vi "Close.vi"(8 "error in (no error)":errorcluster, 11 "KNF Settings":T1={"VISA resource name"="", "Simulated?"=TRUE}) -> (0 "error out":errorcluster, 1 "Connection Error":bool, 3 "KNF Settings":T1={"VISA resource name"="", "Simulated?"=TRUE})   [LabVIEW 2018, in "KNF SIMDOS.lvlib"]
uses:
  KNF SIMDOS.lvlib
  Settings Cluster plus SIMDOS.ctl
  <vilib>/KNF LAB/Driver S/Lvlib/SIMLAB_driver_lvclass/SIMLAB_driver.lvclass
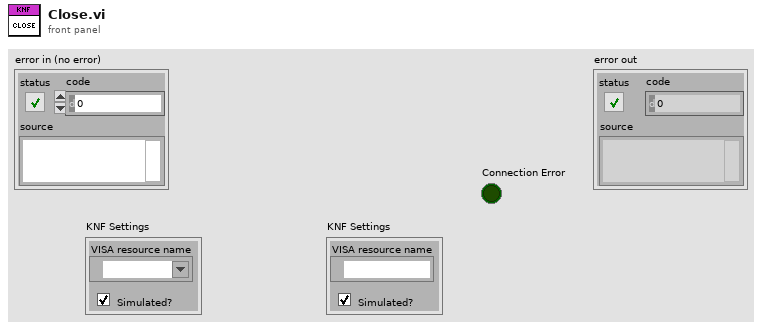
[diagram p1: front panel]
types:
  T1 = typedef "KNF SIMDOS.lvlib/Settings Cluster plus SIMDOS.ctl" = cluster{"VISA resource name":refnum<visa-resource-name>, "Simulated?":bool}
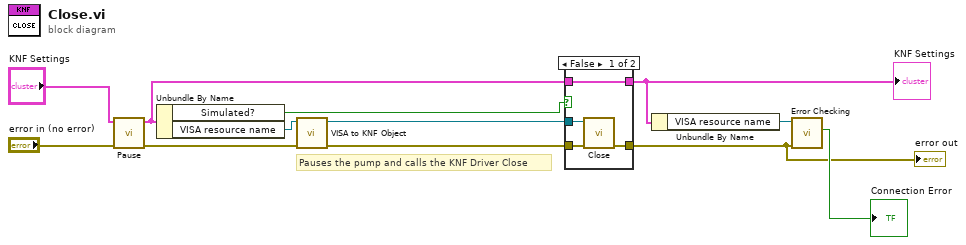
[diagram p0: block diagram]
diagram:
  # "Pauses the pump and calls the KNF Driver Close"
  n1 = call "Pause.vi"("error in (no error)"="error in (no error)", "KNF Settings"="KNF Settings") -> ("error out"=w7:errorcluster, "KNF Settings"=w5:T1)  [unwired: 7 in, 1 out]
  n2 = Unbundle By Name(w5) -> ("Simulated?"=w12:bool, "VISA resource name"=w11:refnum<visa-resource-name>)
  n3 = call "VISA to KNF Object.vi"("error in (no error)"=w7, "VISA resource name"=w11) -> ("error out"=w9:errorcluster, "SIMDOS out"=w10:refnum<class "SIMLAB_driver.lvclass">)  [unwired: 8 in]
  n4 = case shown="False" w12 {
    tunnel: [w15 w18] -> w2
    tunnel: w5 -> [w15 w18]
    tunnel: [w14 w17] -> w3
    tunnel: w9 -> [w13 w17]
    tunnel: w10 -> [w16 _]
    frame False {
      n5 = call <vilib>:"Close.vi"("error in (no error)"=w13, "SIMDOS in"=w16) -> ("error out"=w14:errorcluster)  [unwired: 8 in, 1 out]
    }
    frame True {
    }
  }
  "error out" <- w3
  "KNF Settings" <- w2
  n6 = Unbundle By Name(w2) -> ("VISA resource name"=w1:refnum<visa-resource-name>)
  n7 = call "Error Checking.vi"("error in (no error)"=w3, "VISA resource name"=w1) -> ("Connection Error"=→"Connection Error":bool)  [unwired: 7 in, 2 out]
